vi "Read Wait Time.vi"(8 "error in (no error)":errorcluster, 11 "Wait in":refnum<class "Wait.lvclass">) -> (0 "error out":errorcluster, 2 "Wait Time":dbl, 3 "Wait out":refnum<class "Wait.lvclass">)   [LabVIEW 2015, in "Wait.lvclass"]
uses:
  Wait.lvclass
  Wait.lvclass/Wait.ctl
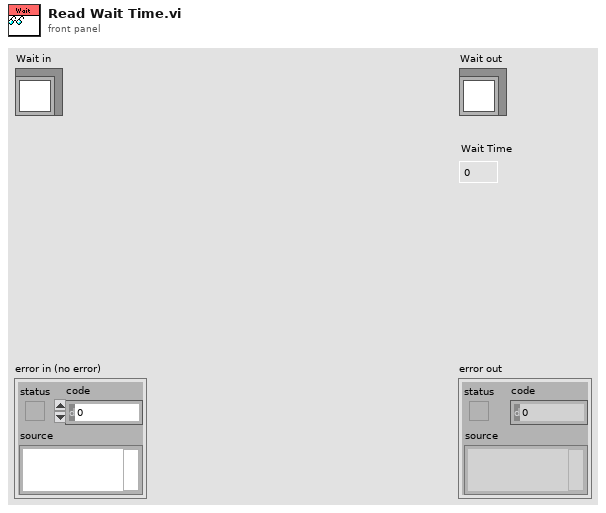
[diagram p1: front panel]
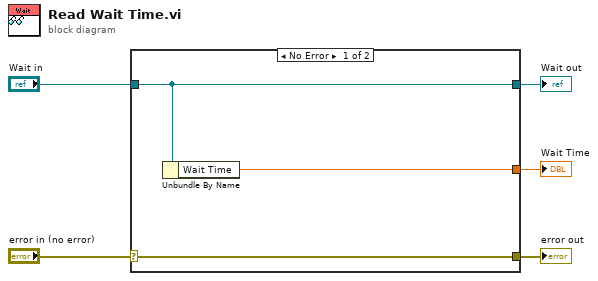
[diagram p0: block diagram]
diagram:
  n1 = case shown="No Error" "error in (no error)" {
    selector: "error in (no error)" -> [w8 w9]
    tunnel: [w8 w9] -> w4
    tunnel: [w7 w10] -> w2
    tunnel: "Wait in" -> [w7 w10]
    tunnel: [w6 _] -> w1
    frame No Error {
      n2 = Unbundle By Name(w7) -> ("Wait Time"=w6:dbl)
    }
    frame Error {
    }
  }
  "error out" <- w4
  "Wait out" <- w2
  "Wait Time" <- w1
